vi "log analysis_gps.vi"() -> ()   [LabVIEW 2018] (continued)
status\tnormal 0 27.800000 0 0\trobot status\t0.680194\t-3.259887\t9.836300\t-0.786931\t0.220983\t9.744504\t0.000000\t0.000000\n\t\n15:54:55.1\tlog_raw\tgps_raw\t#INSPVAXA,USB3,0,53.0,FINESTEERING,2107,284104.050,02000000,471d,15824;INS_ALIGNMENT_COMPLETE,INS_RTKFIXED,37.37010082408,126.72084278410,9.8363,22.3000,-0.0077,0.0002,0.0002,-0.786930858,0.220983047,80.255496235,0.2109,0.1616,0.2842,0.0344,0.0343,0.0312,0.0727,0.0733,4.8905,0f000005,0*84218c18\n\tsystem status\tnormal 0 27.800000 0 0\trobot status\t0.680194\t-3.259887\t9.836300\t-0.786931\t0.220983\t9.744504\t0.000000\t0.000000\n\t\n15:54:55.6\tlog_raw\tgps_raw\t#INSPVAXA,USB3,0,53.0,FINESTEERING,2107,284104.050,02000000,471d,15824;INS_ALIGNMENT_COMPLETE,INS_RTKFIXED,37.37010082408,126.72084278410,9.8363,22.3000,-0.0077,0.0002,0.0002,-0.786930858,0.220983047,80.255496235,0.2109,0.1616,0.2842,0.0344,0.0343,0.0312,0.0727,0.0733,4.8905,0f000005,0*84218c18\n\tsystem status\tnormal 0 27.800000 0 0\trobot status\t0.680194\t-3.259887\t9.836300\t-0.786931\t0.220983\t9.744504\t0.000000\t0.000000\n\t\n15:54:56.1\tlog_raw\tgps_raw\t#INSPVAXA,USB3,0,53.0,FINESTEERING,2107,284104.050,02000000,471d,15824;INS_ALIGNMENT_COMPLETE,INS_RTKFIXED,37.37010082408,126.72084278410,9.8363,22.3000,-0.0077,0.0002,0.0002,-0.786930858,0.220983047,80.255496235,0.2109,0.1616,0.2842,0.0344,0.0343,0.0312,0.0727,0.0733,4.8905,0f000005,0*84218c18\n\tsystem status\tnormal 0 27.800000 0 0\trobot status\t0.680194\t-3.259887\t9.836300\t-0.786931\t0.220983\t9.744504\t0.000000\t0.000000\n\t\n15:54:56.6\tlog_raw\tgps_raw\t#INSPVAXA,USB3,0,53.0,FINESTEERING,2107,284104.050,02000000,471d,15824;INS_ALIGNMENT_COMPLETE,INS_RTKFIXED,37.37010082408,126.72084278410,9.8363,22.3000,-0.0077,0.0002,0.0002,-0.786930858,0.220983047,80.255496235,0.2109,0.1616,0.2842,0.0344,0.0343,0.0312,0.0727,0.0733,4.8905,0f000005,0*84218c18\n\tsystem status\tnormal 0 27.800000 0 0\trobot status\t0.680194\t-3.259887\t9.836300\t-0.786931\t0.220983\t9.744504\t0.000000\t0.000000\n\t\n15:54:57.1\tlog_raw\tgps_raw\t#INSPVAXA,USB3,0,53.0,FINESTEERING,2107,284104.050,02000000,471d,15824;INS_ALIGNMENT_COMPLETE,INS_RTKFIXED,37.37010082408,126.72084278410,9.8363,22.3000,-0.0077,0.0002,0.0002,-0.786930858,0.220983047,80.255496235,0.2109,0.1616,0.2842,0.0344,0.0343,0.0312,0.0727,0.0733,4.8905,0f000005,0*84218c18\n\tsystem status\tnormal 0 27.800000 0 0\trobot status\t0.680194\t-3.259887\t9.836300\t-0.786931\t0.220983\t9.744504\t0.000000\t0.000000\n\t\n15:54:57.6\tlog_raw\tgps_raw\t#INSPVAXA,USB3,0,53.0,FINESTEERING,2107,284104.050,02000000,471d,15824;INS_ALIGNMENT_COMPLETE,INS_RTKFIXED,37.37010082408,126.72084278410,9.8363,22.3000,-0.0077,0.0002,0.0002,-0.786930858,0.220983047,80.255496235,0.2109,0.1616,0.2842,0.0344,0.0343,0.0312,0.0727,0.0733,4.8905,0f000005,0*84218c18\n\tsystem status\tnormal 0 27.800000 0 0\trobot status\t0.680194\t-3.259887\t9.836300\t-0.786931\t0.220983\t9.744504\t0.000000\t0.000000\n\t\n15:54:58.1\tlog_raw\tgps_raw\t#INSPVAXA,USB3,0,53.0,FINESTEERING,2107,284104.050,02000000,471d,15824;INS_ALIGNMENT_COMPLETE,INS_RTKFIXED,37.37010082408,126.72084278410,9.8363,22.3000,-0.0077,0.0002,0.0002,-0.786930858,0.220983047,80.255496235,0.2109,0.1616,0.2842,0.0344,0.0343,0.0312,0.0727,0.0733,4.8905,0f000005,0*84218c18\n\tsystem status\tnormal 0 27.800000 0 0\trobot status\t0.680194\t-3.259887\t9.836300\t-0.786931\t0.220983\t9.744504\t0.000000\t0.000000\n\t\n15:54:58.6\tlog_raw\tgps_raw\t#INSPVAXA,USB3,0,53.0,FINESTEERING,2107,284104.050,02000000,471d,15824;INS_ALIGNMENT_COMPLETE,INS_RTKFIXED,37.37010082408,126.72084278410,9.8363,22.3000,-0.0077,0.0002,0.0002,-0.786930858,0.220983047,80.255496235,0.2109,0.1616,0.2842,0.0344,0.0343,0.0312,0.0727,0.0733,4.8905,0f000005,0*84218c18\n\tsystem status\tnormal 0 27.800000 0 0\trobot status\t0.680194\t-3.259887\t9.836300\t-0.786931\t0.220983\t9.744504\t0.000000\t0.000000\n\t\n15:54:59.1\tlog_raw\tgps_raw\t#INSPVAXA,USB3,0,53.0,FINESTEERING,2107,284104.050,02000000,471d,15824;INS_ALIGNMENT_COMPLETE,INS_RTKFIXED,37.37010082408,126.72084278410,9.8363,22.3000,-0.0077,0.0002,0.0002,-0.786930858,0.220983047,80.255496235,0.2109,0.1616,0.2842,0.0344,0.0343,0.0312,0.0727,0.0733,4.8905,0f000005,0*84218c18\n\tsystem status\tnormal 0 27.800000 0 0\trobot status\t0.680194\t-3.259887\t9.836300\t-0.786931\t0.220983\t9.744504\t0.000000\t0.000000\n\t\n15:54:59.6\tlog_raw\tgps_raw\t#INSPVAXA,USB3,0,53.0,FINESTEERING,2107,284104.050,02000000,471d,15824;INS_ALIGNMENT_COMPLETE,INS_RTKFIXED,37.37010082408,126.72084278410,9.8363,22.3000,-0.0077,0.0002,0.0002,-0.786930858,0.220983047,80.255496235,0.2109,0.1616,0.2842,0.0344,0.0343,0.0312,0.0727,0.0733,4.8905,0f000005,0*84218c18\n\tsystem status\tnormal 0 27.800000 0 0\trobot status\t0.680194\t-3.259887\t9.836300\t-0.786931\t0.220983\t9.744504\t0.000000\t0.000000\n\t\n15:55:00.1\tlog_raw\tgps_raw\t#INSPVAXA,USB3,0,53.0,FINESTEERING,2107,284104.050,02000000,471d,15824;INS_ALIGNMENT_COMPLETE,INS_RTKFIXED,37.37010082408,126.72084278410,9.8363,22.3000,-0.0077,0.0002,0.0002,-0.786930858,0.220983047,80.255496235,0.2109,0.1616,0.2842,0.0344,0.0343,0.0312,0.0727,0.0733,4.8905,0f000005,0*84218c18\n\tsystem status\tnormal 0 27.800000 0 0\trobot status\t0.680194\t-3.259887\t9.836300\t-0.786931\t0.220983\t9.744504\t0.000000\t0.000000\n\t\n15:55:00.6\tlog_raw\tgps_raw\t#INSPVAXA,USB3,0,53.0,FINESTEERING,2107,284104.050,02000000,471d,15824;INS_ALIGNMENT_COMPLETE,INS_RTKFIXED,37.37010082408,126.72084278410,9.8363,22.3000,-0.0077,0.0002,0.0002,-0.786930858,0.220983047,80.255496235,0.2109,0.1616,0.2842,0.0344,0.0343,0.0312,0.0727,0.0733,4.8905,0f000005,0*84218c18\n\tsystem status\tnormal 0 27.800000 0 0\trobot status\t0.680194\t-3.259887\t9.836300\t-0.786931\t0.220983\t9.744504\t0.000000\t0.000000\n\t\n15:55:01.1\tlog_raw\tgps_raw\t#INSPVAXA,USB3,0,53.0,FINESTEERING,2107,284104.050,02000000,471d,15824;INS_ALIGNMENT_COMPLETE,INS_RTKFIXED,37.37010082408,126.72084278410,9.8363,22.3000,-0.0077,0.0002,0.0002,-0.786930858,0.220983047,80.255496235,0.2109,0.1616,0.2842,0.0344,0.0343,0.0312,0.0727,0.0733,4.8905,0f000005,0*84218c18\n\tsystem status\tnormal 0 27.800000 0 0\trobot status\t0.680194\t-3.259887\t9.836300\t-0.786931\t0.220983\t9.744504\t0.000000\t0.000000\n\t\n15:55:01.6\tlog_raw\tgps_raw\t#INSPVAXA,USB3,0,53.0,FINESTEERING,2107,284104.050,02000000,471d,15824;INS_ALIGNMENT_COMPLETE,INS_RTKFIXED,37.37010082408,126.72084278410,9.8363,22.3000,-0.0077,0.0002,0.0002,-0.786930858,0.220983047,80.255496235,0.2109,0.1616,0.2842,0.0344,0.0343,0.0312,0.0727,0.0733,4.8905,0f000005,0*84218c18\n\tsystem status\tnormal 0 27.800000 0 0\trobot status\t0.680194\t-3.259887\t9.836300\t-0.786931\t0.220983\t9.744504\t0.000000\t0.000000\n\t\n15:55:02.1\tlog_raw\tgps_raw\t#INSPVAXA,USB3,0,53.0,FINESTEERING,2107,284104.050,02000000,471d,15824;INS_ALIGNMENT_COMPLETE,INS_RTKFIXED,37.37010082408,126.72084278410,9.8363,22.3000,-0.0077,0.0002,0.0002,-0.786930858,0.220983047,80.255496235,0.2109,0.1616,0.2842,0.0344,0.0343,0.0312,0.0727,0.0733,4.8905,0f000005,0*84218c18\n\tsystem status\tnormal 0 27.800000 0 0\trobot status\t0.680194\t-3.259887\t9.836300\t-0.786931\t0.220983\t9.744504\t0.000000\t0.000000\n\t\n15:55:02.6\tlog_raw\tgps_raw\t#INSPVAXA,USB3,0,53.0,FINESTEERING,2107,284104.050,02000000,471d,15824;INS_ALIGNMENT_COMPLETE,INS_RTKFIXED,37.37010082408,126.72084278410,9.8363,22.3000,-0.0077,0.0002,0.0002,-0.786930858,0.220983047,80.255496235,0.2109,0.1616,0.2842,0.0344,0.0343,0.0312,0.0727,0.0733,4.8905,0f000005,0*84218c18\n\tsystem status\tnormal 0 27.800000 0 0\trobot status\t0.680194\t-3.259887\t9.836300\t-0.786931\t0.220983\t9.744504\t0.000000\t0.000000\n\t\n15:55:03.1\tlog_raw\tgps_raw\t#INSPVAXA,USB3,0,53.0,FINESTEERING,2107,284104.050,02000000,471d,15824;INS_ALIGNMENT_COMPLETE,INS_RTKFIXED,37.37010082408,126.72084278410,9.8363,22.3000,-0.0077,0.0002,0.0002,-0.786930858,0.220983047,80.255496235,0.2109,0.1616,0.2842,0.0344,0.0343,0.0312,0.0727,0.0733,4.8905,0f000005,0*84218c18\n\tsystem status\tnormal 0 27.800000 0 0\trobot status\t0.680194\t-3.259887\t9.836300\t-0.786931\t0.220983\t9.744504\t0.000000\t0.000000\n\t\n15:55:03.6\tlog_raw\tgps_raw\t#INSPVAXA,USB3,0,53.0,FINESTEERING,2107,284104.050,02000000,471d,15824;INS_ALIGNMENT_COMPLETE,INS_RTKFIXED,37.37010082408,126.72084278410,9.8363,22.3000,-0.0077,0.0002,0.0002,-0.786930858,0.220983047,80.255496235,0.2109,0.1616,0.2842,0.0344,0.0343,0.0312,0.0727,0.0733,4.8905,0f000005,0*84218c18\n\tsystem status\tnormal 0 27.800000 0 0\trobot status\t0.680194\t-3.259887\t9.836300\t-0.786931\t0.220983\t9.744504\t0.000000\t0.000000\n\t\n15:55:04.1\tlog_raw\tgps_raw\t#INSPVAXA,USB3,0,53.0,FINESTEERING,2107,284104.050,02000000,471d,15824;INS_ALIGNMENT_COMPLETE,INS_RTKFIXED,37.37010082408,126.72084278410,9.8363,22.3000,-0.0077,0.0002,0.0002,-0.786930858,0.220983047,80.255496235,0.2109,0.1616,0.2842,0.0344,0.0343,0.0312,0.0727,0.0733,4.8905,0f000005,0*84218c18\n\tsystem status\tnormal 0 27.800000 0 0\trobot status\t0.680194\t-3.259887\t9.836300\t-0.786931\t0.220983\t9.744504\t0.000000\t0.000000\n\t\n15:55:04.6\tlog_raw\tgps_raw\t#INSPVAXA,USB3,0,53.0,FINESTEERING,2107,284104.050,02000000,471d,15824;INS_ALIGNMENT_COMPLETE,INS_RTKFIXED,37.37010082408,126.72084278410,9.8363,22.3000,-0.0077,0.0002,0.0002,-0.786930858,0.220983047,80.255496235,0.2109,0.1616,0.2842,0.0344,0.0343,0.0312,0.0727,0.0733,4.8905,0f000005,0*84218c18\n\tsystem status\tnormal 0 27.800000 0 0\trobot status\t0.680194\t-3.259887\t9.836300\t-0.786931\t0.220983\t9.744504\t0.000000\t0.000000\n\t\n15:55:05.1\tlog_raw\tgps_raw\t#INSPVAXA,USB3,0,53.0,FINESTEERING,2107,284104.050,02000000,471d,15824;INS_ALIGNMENT_COMPLETE,INS_RTKFIXED,37.37010082408,126.72084278410,9.8363,22.3000,-0.0077,0.0002,0.0002,-0.786930858,0.220983047,80.255496235,0.2109,0.1616,0.2842,0.0344,0.0343,0.0312,0.0727,0.0733,4.8905,0f000005,0*84218c18\n\tsystem status\tnormal 0 27.800000 0 0\trobot status\t0.680194\t-3.259887\t9.836300\t-0.786931\t0.220983\t9.744504\t0.000000\t0.000000\n\t\n15:55:05.6\tlog_raw\tgps_raw\t#INSPVAXA,USB3,0,53.0,FINESTEERING,2107,284104.050,02000000,471d,15824;INS_ALIGNMENT_COMPLETE,INS_RTKFIXED,37.37010082408,126.72084278410,9.8363,22.3000,-0.0077,0.0002,0.0002,-0.786930858,0.220983047,80.255496235,0.2109,0.1616,0.2842,0.0344,0.0343,0.0312,0.0727,0.0733,4.8905,0f000005,0*84218c18\n\tsystem status\tnormal 0 27.800000 0 0\trobot status\t0.680194\t-3.259887\t9.836300\t-0.786931\t0.220983\t9.744504\t0.000000\t0.000000\n\t\n15:55:06.1\tlog_raw\tgps_raw\t#INSPVAXA,USB3,0,53.0,FINESTEERING,2107,284104.050,02000000,471d,15824;INS_ALIGNMENT_COMPLETE,INS_RTKFIXED,37.37010082408,126.72084278410,9.8363,22.3000,-0.0077,0.0002,0.0002,-0.786930858,0.220983047,80.255496235,0.2109,0.1616,0.2842,0.0344,0.0343,0.0312,0.0727,0.0733,4.8905,0f000005,0*84218c18\n\tsystem status\tnormal 0 27.800000 0 0\trobot status\t0.680194\t-3.259887\t9.836300\t-0.786931\t0.220983\t9.744504\t0.000000\t0.000000\n\t\n15:55:06.6\tlog_raw\tgps_raw\t#INSPVAXA,USB3,0,53.0,FINESTEERING,2107,284104.050,02000000,471d,15824;INS_ALIGNMENT_COMPLETE,INS_RTKFIXED,37.37010082408,126.72084278410,9.8363,22.3000,-0.0077,0.0002,0.0002,-0.786930858,0.220983047,80.255496235,0.2109,0.1616,0.2842,0.0344,0.0343,0.0312,0.0727,0.0733,4.8905,0f000005,0*84218c18\n\tsystem status\tnormal 0 27.800000 0 0\trobot status\t0.680194\t-3.259887\t9.836300\t-0.786931\t0.220983\t9.744504\t0.000000\t0.000000\n\t\n15:55:07.1\tlog_raw\tgps_raw\t#INSPVAXA,USB3,0,53.0,FINESTEERING,2107,284104.050,02000000,471d,15824;INS_ALIGNMENT_COMPLETE,INS_RTKFIXED,37.37010082408,126.72084278410,9.8363,22.3000,-0.0077,0.0002,0.0002,-0.786930858,0.220983047,80.255496235,0.2109,0.1616,0.2842,0.0344,0.0343,0.0312,0.0727,0.0733,4.8905,0f000005,0*84218c18\n\tsystem status\tnormal 0 27.800000 0 0\trobot status\t0.680194\t-3.259887\t9.836300\t-0.786931\t0.220983\t9.744504\t0.000000\t0.000000\n\t\n15:55:07.6\tlog_raw\tgps_raw\t#INSPVAXA,USB3,0,53.0,FINESTEERING,2107,284104.050,02000000,471d,15824;INS_ALIGNMENT_COMPLETE,INS_RTKFIXED,37.37010082408,126.72084278410,9.8363,22.3000,-0.0077,0.0002,0.0002,-0.786930858,0.220983047,80.255496235,0.2109,0.1616,0.2842,0.0344,0.0343,0.0312,0.0727,0.0733,4.8905,0f000005,0*84218c18\n\tsystem status\tnormal 0 27.800000 0 0\trobot status\t0.680194\t-3.259887\t9.836300\t-0.786931\t0.220983\t9.744504\t0.000000\t0.000000\n\t\n15:55:08.1\tlog_raw\tgps_raw\t#INSPVAXA,USB3,0,53.0,FINESTEERING,2107,284104.050,02000000,471d,15824;INS_ALIGNMENT_COMPLETE,INS_RTKFIXED,37.37010082408,126.72084278410,9.8363,22.3000,-0.0077,0.0002,0.0002,-0.786930858,0.220983047,80.255496235,0.2109,0.1616,0.2842,0.0344,0.0343,0.0312,0.0727,0.0733,4.8905,0f000005,0*84218c18\n\tsystem status\tnormal 0 27.800000 0 0\trobot status\t0.680194\t-3.259887\t9.836300\t-0.786931\t0.220983\t9.744504\t0.000000\t0.000000\n\t\n15:55:08.6\tlog_raw\tgps_raw\t#INSPVAXA,USB3,0,53.0,FINESTEERING,2107,284104.050,02000000,471d,15824;INS_ALIGNMENT_COMPLETE,INS_RTKFIXED,37.37010082408,126.72084278410,9.8363,22.3000,-0.0077,0.0002,0.0002,-0.786930858,0.220983047,80.255496235,0.2109,0.1616,0.2842,0.0344,0.0343,0.0312,0.0727,0.0733,4.8905,0f000005,0*84218c18\n\tsystem status\tnormal 0 27.800000 0 0\trobot status\t0.680194\t-3.259887\t9.836300\t-0.786931\t0.220983\t9.744504\t0.000000\t0.000000\n\t\n15:55:09.1\tlog_raw\tgps_raw\t#INSPVAXA,USB3,0,53.0,FINESTEERING,2107,284104.050,02000000,471d,15824;INS_ALIGNMENT_COMPLETE,INS_RTKFIXED,37.37010082408,126.72084278410,9.8363,22.3000,-0.0077,0.0002,0.0002,-0.786930858,0.220983047,80.255496235,0.2109,0.1616,0.2842,0.0344,0.0343,0.0312,0.0727,0.0733,4.8905,0f000005,0*84218c18\n\tsystem status\tnormal 0 27.800000 0 0\trobot status\t0.680194\t-3.259887\t9.836300\t-0.786931\t0.220983\t9.744504\t0.000000\t0.000000\n\t\n15:55:09.6\tlog_raw\tgps_raw\t#INSPVAXA,USB3,0,53.0,FINESTEERING,2107,284104.050,02000000,471d,15824;INS_ALIGNMENT_COMPLETE,INS_RTKFIXED,37.37010082408,126.72084278410,9.8363,22.3000,-0.0077,0.0002,0.0002,-0.786930858,0.220983047,80.255496235,0.2109,0.1616,0.2842,0.0344,0.0343,0.0312,0.0727,0.0733,4.8905,0f000005,0*84218c18\n\tsystem status\tnormal 0 27.800000 0 0\trobot status\t0.680194\t-3.259887\t9.836300\t-0.786931\t0.220983\t9.744504\t0.000000\t0.000000\n\t\n15:55:10.1\tlog_raw\tgps_raw\t#INSPVAXA,USB3,0,53.0,FINESTEERING,2107,284104.050,02000000,471d,15824;INS_ALIGNMENT_COMPLETE,INS_RTKFIXED,37.37010082408,126.72084278410,9.8363,22.3000,-0.0077,0.0002,0.0002,-0.786930858,0.220983047,80.255496235,0.2109,0.1616,0.2842,0.0344,0.0343,0.0312,0.0727,0.0733,4.8905,0f000005,0*84218c18\n\tsystem status\tnormal 0 27.800000 0 0\trobot status\t0.680194\t-3.259887\t9.836300\t-0.786931\t0.220983\t9.744504\t0.000000\t0.000000\n\t\n15:55:10.6\tlog_raw\tgps_raw\t#INSPVAXA,USB3,0,53.0,FINESTEERING,2107,284104.050,02000000,471d,15824;INS_ALIGNMENT_COMPLETE,INS_RTKFIXED,37.37010082408,126.72084278410,9.8363,22.3000,-0.0077,0.0002,0.0002,-0.786930858,0.220983047,80.255496235,0.2109,0.1616,0.2842,0.0344,0.0343,0.0312,0.0727,0.0733,4.8905,0f000005,0*84218c18\n\tsystem status\tnormal 0 27.800000 0 0\trobot status\t0.680194\t-3.259887\t9.836300\t-0.786931\t0.220983\t9.744504\t0.000000\t0.000000\n\t\n"
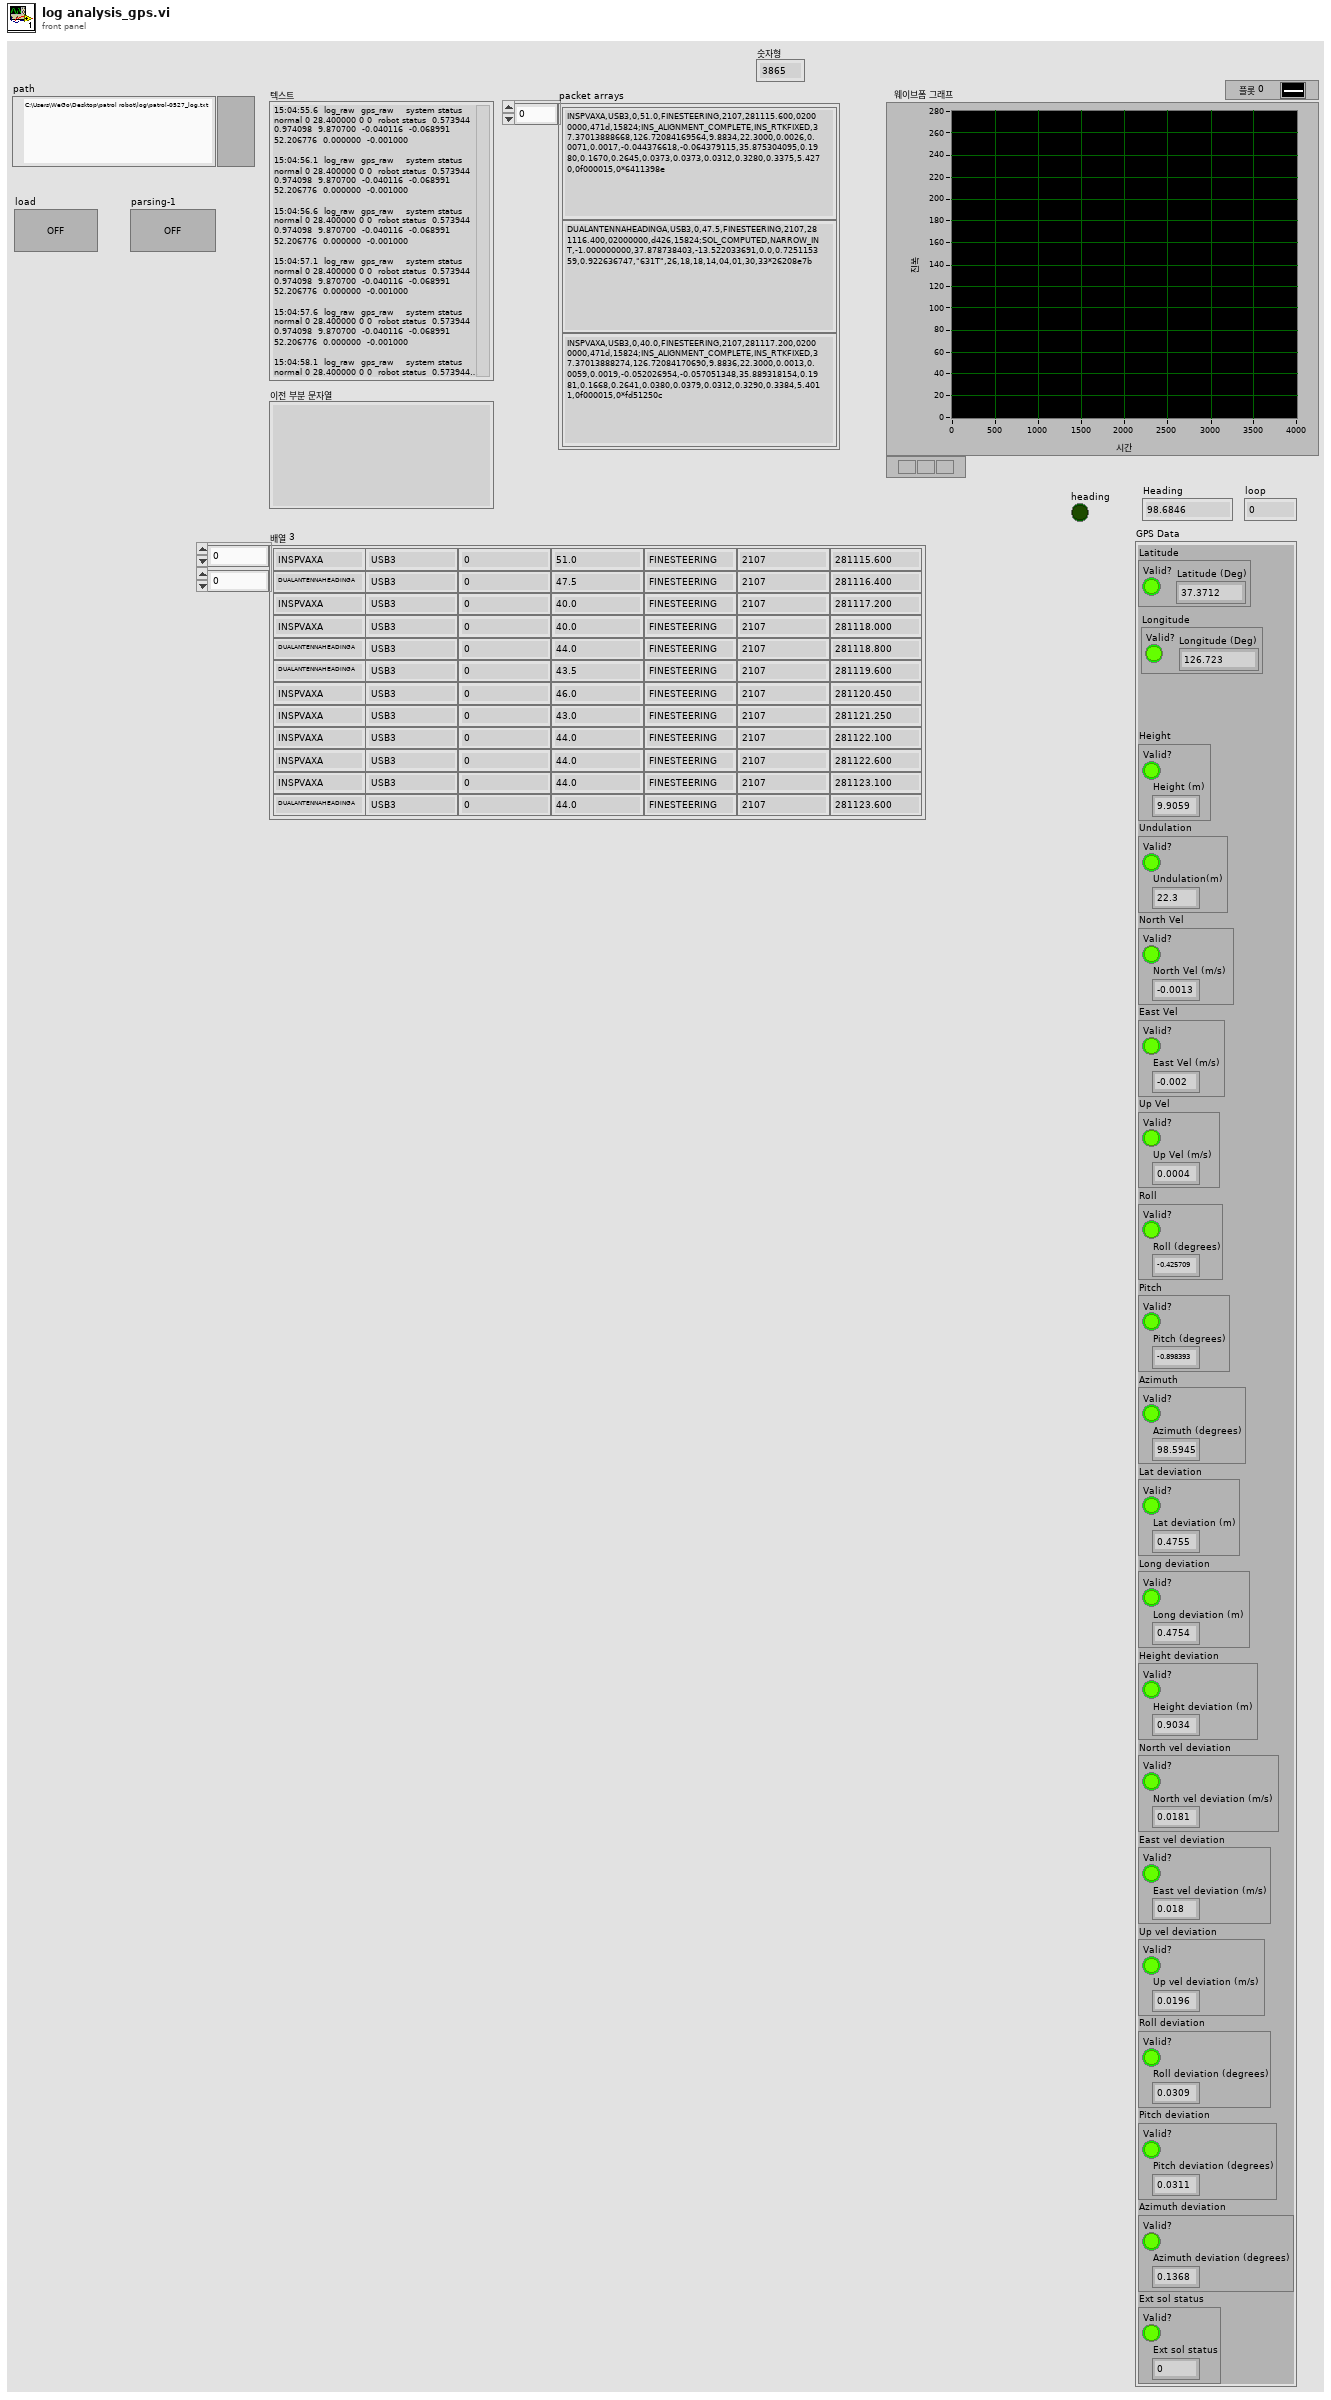
[diagram p1: front panel]
types:
  T1 = cluster{"Latitude":cluster{"Valid?":bool, "Latitude (Deg)":dbl}, "Longitude":cluster{"Valid?":bool, "Longitude (Deg)":dbl}, "Height":cluster{"Valid?":bool, "Height (m)":dbl}, "Undulation":cluster{"Valid?":bool, "Undulation(m)":dbl}, "North Vel":cluster{"Valid?":bool, "North Vel (m/s)":dbl}, "East Vel":cluster{"Valid?":bool, "East Vel (m/s)":dbl}, "Up Vel":cluster{"Valid?":bool, "Up Vel (m/s)":dbl}, "Roll":cluster{"Valid?":bool, "Roll (degrees)":dbl}, "Pitch":cluster{"Valid?":bool, "Pitch (degrees)":dbl}, "Azimuth":cluster{"Valid?":bool, "Azimuth (degrees)":dbl}, "Lat deviation":cluster{"Valid?":bool, "Lat deviation (m)":dbl}, "Long deviation":cluster{"Valid?":bool, "Long deviation (m)":dbl}, "Height deviation":cluster{"Valid?":bool, "Height deviation (m)":dbl}, "North vel deviation":cluster{"Valid?":bool, "North vel deviation (m/s)":dbl}, "East vel deviation":cluster{"Valid?":bool, "East vel deviation (m/s)":dbl}, "Up vel deviation":cluster{"Valid?":bool, "Up vel deviation (m/s)":dbl}, "Roll deviation":cluster{"Valid?":bool, "Roll deviation (degrees)":dbl}, "Pitch deviation":cluster{"Valid?":bool, "Pitch deviation (degrees)":dbl}, "Azimuth deviation":cluster{"Valid?":bool, "Azimuth deviation (degrees)":dbl}, "Ext sol status":cluster{"Valid?":bool, "Ext sol status":dbl}}
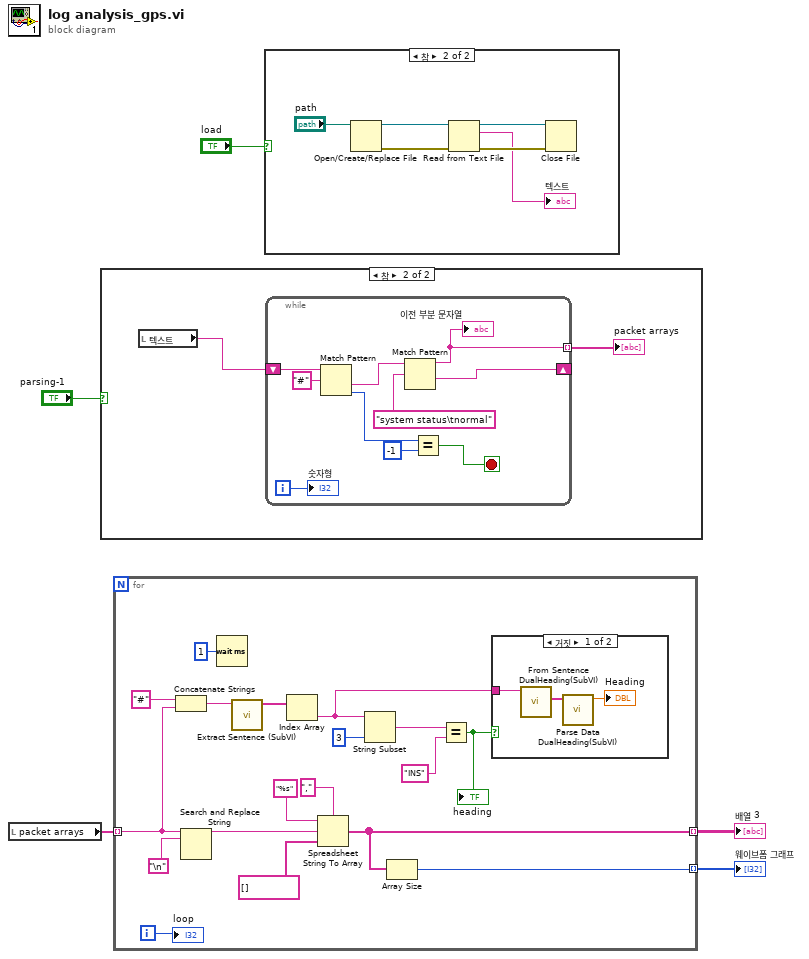
[diagram p0: block diagram]
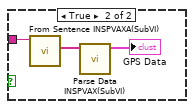
[diagram p2: hidden frame]
diagram:
  n1 = local read "packet arrays"() -> (w3:string[])
  n2 = case shown="참" "parsing-1" {
    frame False {
    }
    frame True {
      n3 = local read "텍스트"() -> (w7:string)
      n4 = while {
        tunnel: [w8] -> w6 mode=indexing
        shift-right: [w9] -> _
        shift-left: w7 -> [w17]
        i -> [w10]
        stop <- w11 stop-if-true
        n5 = Match Pattern(string=w17, regular expression="#" ("정규식")) -> (after substring=w14:string, offset past match=w13:i32)  [unwired: 1 in, 2 out]
        n6 = Match Pattern(string=w14, regular expression="system status\tnormal" ("정규식")) -> (before substring=w8:string, after substring=w9:string)  [unwired: 1 in, 2 out]
        "이전 부분 문자열" <- w8
        n7 = Equal?(x=w13, y=-1) -> (x = y?=w11:bool)
        "숫자형" <- w10
      }
      "packet arrays" <- w6
    }
  }
  n8 = for {
    tunnel: w3 -> [w22] mode=indexing
    tunnel: [w30] -> w2 mode=indexing
    tunnel: [w29] -> w1 mode=indexing
    i -> [w24]
    n9 = Concatenate Strings("#" ("문자열"), w22) -> (w18:string)
    n10 = Search and Replace String(input string=w22, search string="\n") -> (result string=w32:string)  [unwired: 6 in, 3 out]
    n11 = Wait (ms)(milliseconds to wait=u32 1 ("대기 시간 (ms)")) -> ()  [unwired: 1 out]
    n12 = call "Extract Sentence (SubVI).vi"("raw sentences"=w18) -> ("extract sentences"=w25:string[])  [unwired: 10 in]
    n13 = Index Array(array=w25) -> (element=w27:string)  [unwired: 1 in]
    n14 = Spreadsheet String To Array(delimiter (Tab)="," ("구분 문자 (탭)"), format string="%s" ("포맷 문자열"), spreadsheet string=w32, array type (2D Dbl)=string[] []) -> (array=w30:string[])
    n15 = String Subset(string=w27, length (rest)=3 ("길이(나머지)")) -> (substring=w20:string)  [unwired: 1 in]
    n16 = Array Size(array=w30) -> (size(s)=w29:i32)
    n17 = Equal?(x=w20, y="INS" ("x")) -> (x = y?=w28:bool)
    "heading" <- w28
    n18 = case shown="거짓" w28 {
      tunnel: w27 -> [w36 w41]
      frame False {
        n19 = call "From Sentence DualHeading(SubVI).vi"("Extract Sentence"=w36) -> ("Parse Data Array"=w38:string[])  [unwired: 9 in, 1 out]
        n20 = call "Parse Data DualHeading(SubVI).vi"("Parse Data Array"=w38) -> ("Heading"=→"Heading":dbl)  [unwired: 10 in]
      }
      frame True {
        n21 = call "From Sentence INSPVAXA(SubVI).vi"("Extract Sentence"=w41) -> ("Parse Data Array"=w40:string[])  [unwired: 9 in, 1 out]
        n22 = call "Parse Data INSPVAX(SubVI).vi"("Parse Data Array"=w40) -> ("output cluster"=→"GPS Data":T1)  [unwired: 10 in]
      }
    }
    "loop" <- w24
  }
  "배열 3" <- w2
  "웨이브폼 그래프" <- w1
  n23 = case shown="참" "load" {
    frame False {
    }
    frame True {
      n24 = Open/Create/Replace File(file path (use dialog)="path") -> (refnum out=w47:refnum<file>, error out=w46:errorcluster)  [unwired: 5 in, 1 out]
      n25 = Read from Text File(file (use dialog)=w47, error in=w46) -> (refnum out=w44:refnum<file>, text=→"텍스트":string, error out=w45:errorcluster)  [unwired: 2 in, 1 out]
      n26 = Close File(refnum=w44, error in=w45) -> ()  [unwired: 2 out]
    }
  }
